vi "Read Sim. Command .vi"(8 "error in (no error)":errorcluster, 11 "Simulated uC in":refnum<class "Simulated uC.lvclass">) -> (0 "error out":errorcluster, 2 "Sim. Command":variant, 3 "Simulated uC out":refnum<class "Simulated uC.lvclass">)   [LabVIEW 2019, in "Simulated uC.lvclass"]
uses:
  Simulated uC.lvclass
  Simulated uC.lvclass/Simulated uC.ctl
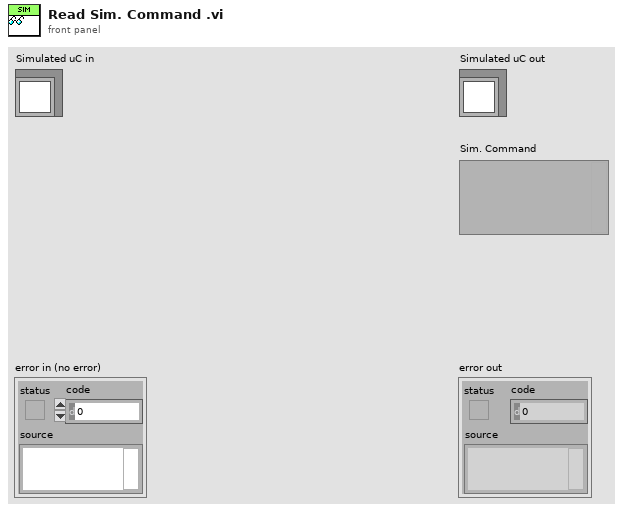
[diagram p1: front panel]
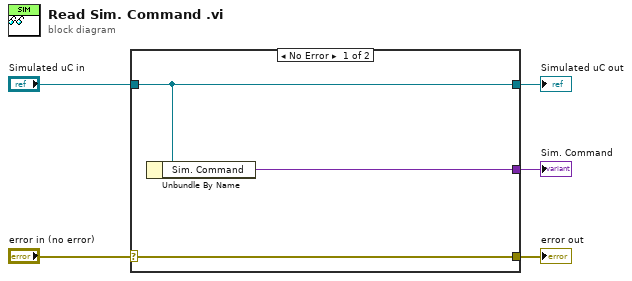
[diagram p0: block diagram]
diagram:
  n1 = case shown="No Error" "error in (no error)" {
    selector: "error in (no error)" -> [w8 w9]
    tunnel: [w8 w9] -> w4
    tunnel: [w7 w10] -> w2
    tunnel: "Simulated uC in" -> [w7 w10]
    tunnel: [w6 _] -> w1
    frame No Error {
      n2 = Unbundle By Name(w7) -> ("Sim. Command"=w6:variant)
    }
    frame Error {
    }
  }
  "error out" <- w4
  "Simulated uC out" <- w2
  "Sim. Command" <- w1
